vi "XML Script - Tunnels.vi"(0 "# of Tunnels":i32, 3 "default":bool, 4 "location":T1, 6 "name":string, 9 "prefix (name)":string) -> (5 "name(s)":string[](array[string]), 7 "XML":string)   [LabVIEW 2017]
uses:
  <vilib>/_script/XML Scripting/Structure Location.ctl
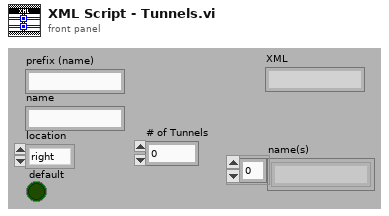
[diagram p1: front panel]
types:
  T1 = typedef "Structure Location.ctl" = enum16{"right", "left", "top", "bottom"}
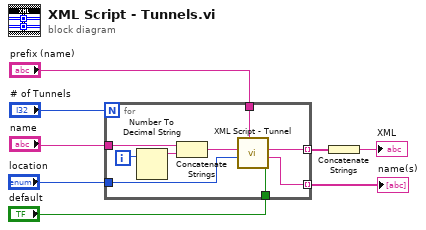
[diagram p0: block diagram]
diagram:
  n1 = for {
    N: "# of Tunnels" -> [_]
    tunnel: [w17] -> w8 mode=indexing
    tunnel: "prefix (name)" -> [w16]
    tunnel: [w15] -> w2 mode=indexing
    tunnel: "location" -> [w11]
    tunnel: "name" -> [w10]
    tunnel: "default" -> [w9]
    i -> [w14]
    n2 = Number To Decimal String(number=w14) -> (decimal integer string=w12:string)  [unwired: 1 out]
    n3 = Concatenate Strings(w10, w12) -> (w13:string)
    n4 = call <vilib>:"XML Script - Tunnel.vi"("default"=w9, "location"=w11, "name"=w13, "prefix (name)"=w16) -> ("name (wire source)"=w15:string, "XML Script Command - Tunnel"=w17:string)  [unwired: 3 in, 3 out]
  }
  "name(s)" <- w2
  n5 = Concatenate Strings(w8) -> (→"XML":string)
